vi "Untitled 1.vi"() -> ()   [LabVIEW 2018]
panel:
  out "x+y":dbl
  in  "y":dbl
  in  "Numeric":dbl
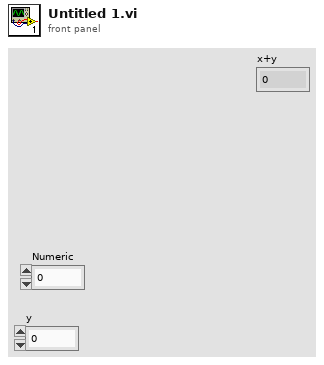
[diagram p1: front panel]
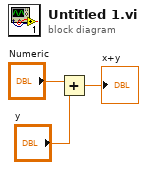
[diagram p0: block diagram]
diagram:
  n1 = Add(x="Numeric", y="y") -> (x+y=→"x+y":dbl)
